vi "Particles_Setting_UI.vi"(4 "ForCalCalculaton In":T1, 6 "Analysis_Setting IN":T2={"PreProcess"=enum."*Algorithm*", "Parameter"=""}, 8 "error in (no error)":errorcluster, 9 "ProjectName":string, 10 "ROI List IN":refnum<vi>, 11 "Vision_Image":T1(plugin-control)) -> (0 "error out":errorcluster, 1 "Cancel?":bool, 2 "TempAnalysisResult":variant, 3 "Analysis_Setting":T2={"PreProcess"=enum."*Algorithm*", "Parameter"=""})   [LabVIEW 2019]
uses:
  Controls/_UI Command Cluster/Particle_UI Command Cluster.ctl
  Controls/Analysis_Type.ctl
  Controls/Analysis_Setting.ctl
  Controls/Particle/Analysis_Particle_Parameter.ctl
  <vilib>/vision/NI_Vision_Development_Module.lvlib
  Controls/V_Analysis_Type.ctl
  <vilib>/vision/Image Controls.llb/IMAQ Image.ctl
  Ctrl/VisionProcessName.ctl
panel:
  in  "Selected Particle":i32=2 min=-1 max=34
  in  "Simulation":bool
  out "Numeric":i32
  in  "Done":bool caption="完成"
  in  "Particle_UI Command":T4(ring)
  in  "Cancel":bool caption="取消"
  in  "ParticleTab":T5(tab)
  in  "MaxParticle":i32=1
  in  "Connectivity 4/8 (8)":bool=TRUE
  out "Selected Particle Report":T6(array[cluster]) {"Orientation" format="%.2f"; "Center of Mass"."Y" format="%.2f"; "Center of Mass"."X" format="%.2f"}
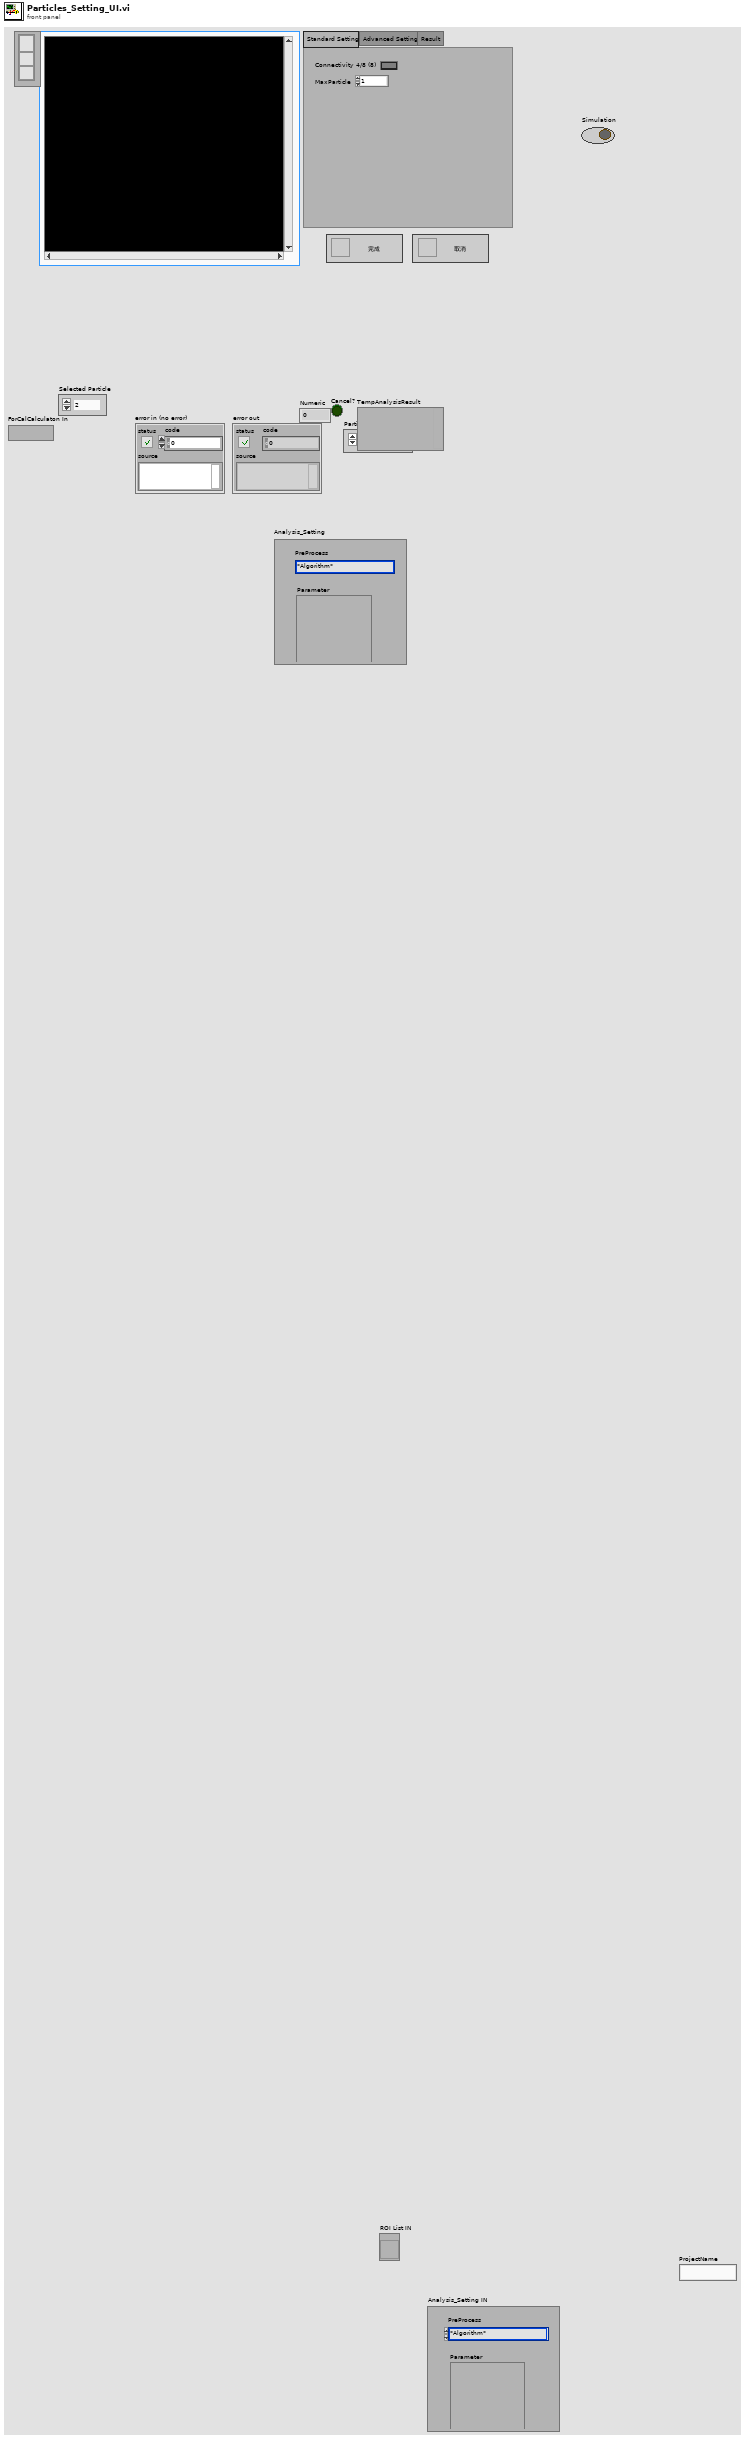
[diagram p1: front panel]
types:
  T1 = typedef "IMAQ Image.ctl" = refnum<image>
  T2 = typedef "Analysis_Setting.ctl" = cluster{"PreProcess":T3, "Parameter":string}
  T3 = typedef "VisionProcessName.ctl" = enum16{"*CamParameter*", "CamAttributes", "*Preprocess*", "CG_Brightness", "C_Plane Extraction", "C_Threshold", "G_Lookup Table", "G_Threshold", "B_Image Inversion", "*Algorithm*", "CG_Histogram", "C_Color Matching", "C_Color Pattern Matching", "G_PatternMatch", "CG_Find Straight Edge", "CG_Adv. Find Straight Edge", "CG_Find Circular Edge", "G_Max Clamp", "G_Clamp (Rake)", "G_Pattern Matching"}
  T4 = enum16{"Initialize", "Done", "Run Algorithm", "Cancel"}
  T5 = enum32{"Standard Setting", "Advanced Setting", "Result"}
  T6 = cluster{"Area":dbl, "Number of Holes":dbl, "Bounding Rect":cluster{"Left":dbl, "Top":dbl, "Right":dbl, "Bottom":dbl}, "Center of Mass":cluster{"X":dbl, "Y":dbl}, "Orientation":dbl, "Dimensions":cluster{"Width":dbl, "Height":dbl}}[]
  T7 = typedef "Particle_UI Command Cluster.ctl" = cluster{"Particle_UI Command":enum16{"Initialize", "Done", "Run Algorithm", "Cancel"}, "Selected Particle":i32, "Snap Simulation Mouse Down":bool, "Connectivity 4/8 (8)":bool, "MaxParticle":i32}
  T8 = typedef "IMAQ Line" = cluster{"Start X":i32, "Start Y":i32, "End X":i32, "End Y":i32}
  T9 = cluster{"Contour Type":u32, "ROI Type":u32, "Points":i32[]}
  T10 = typedef "Image Type" = u32
  T11 = typedef "Analysis_Particle_Parameter.ctl" = cluster{"Selected Particle":i32, "Connectivity 4/8 (8)":bool, "MaxParticle":i32}
  T12 = typedef "Analysis_Type.ctl" = u16
  T13 = typedef "ROI Descriptor" = cluster{"Global Rectangle":i32[], "Contours":cluster{"ID":enum32{"External", "Internal"}, "Type":u32, "Coordinates":i32[]}[]}
  T14 = typedef "Analysis_Setting.ctl" = cluster{"PreProcess":T15, "Parameter":string}
  T15 = typedef "V_Analysis_Type.ctl" = enum16{"None", "C_Color Pattern Matching", "G_PatternMatching", "G_ShapeDectect", "G_GeometricMatch", "B_Area Check"}
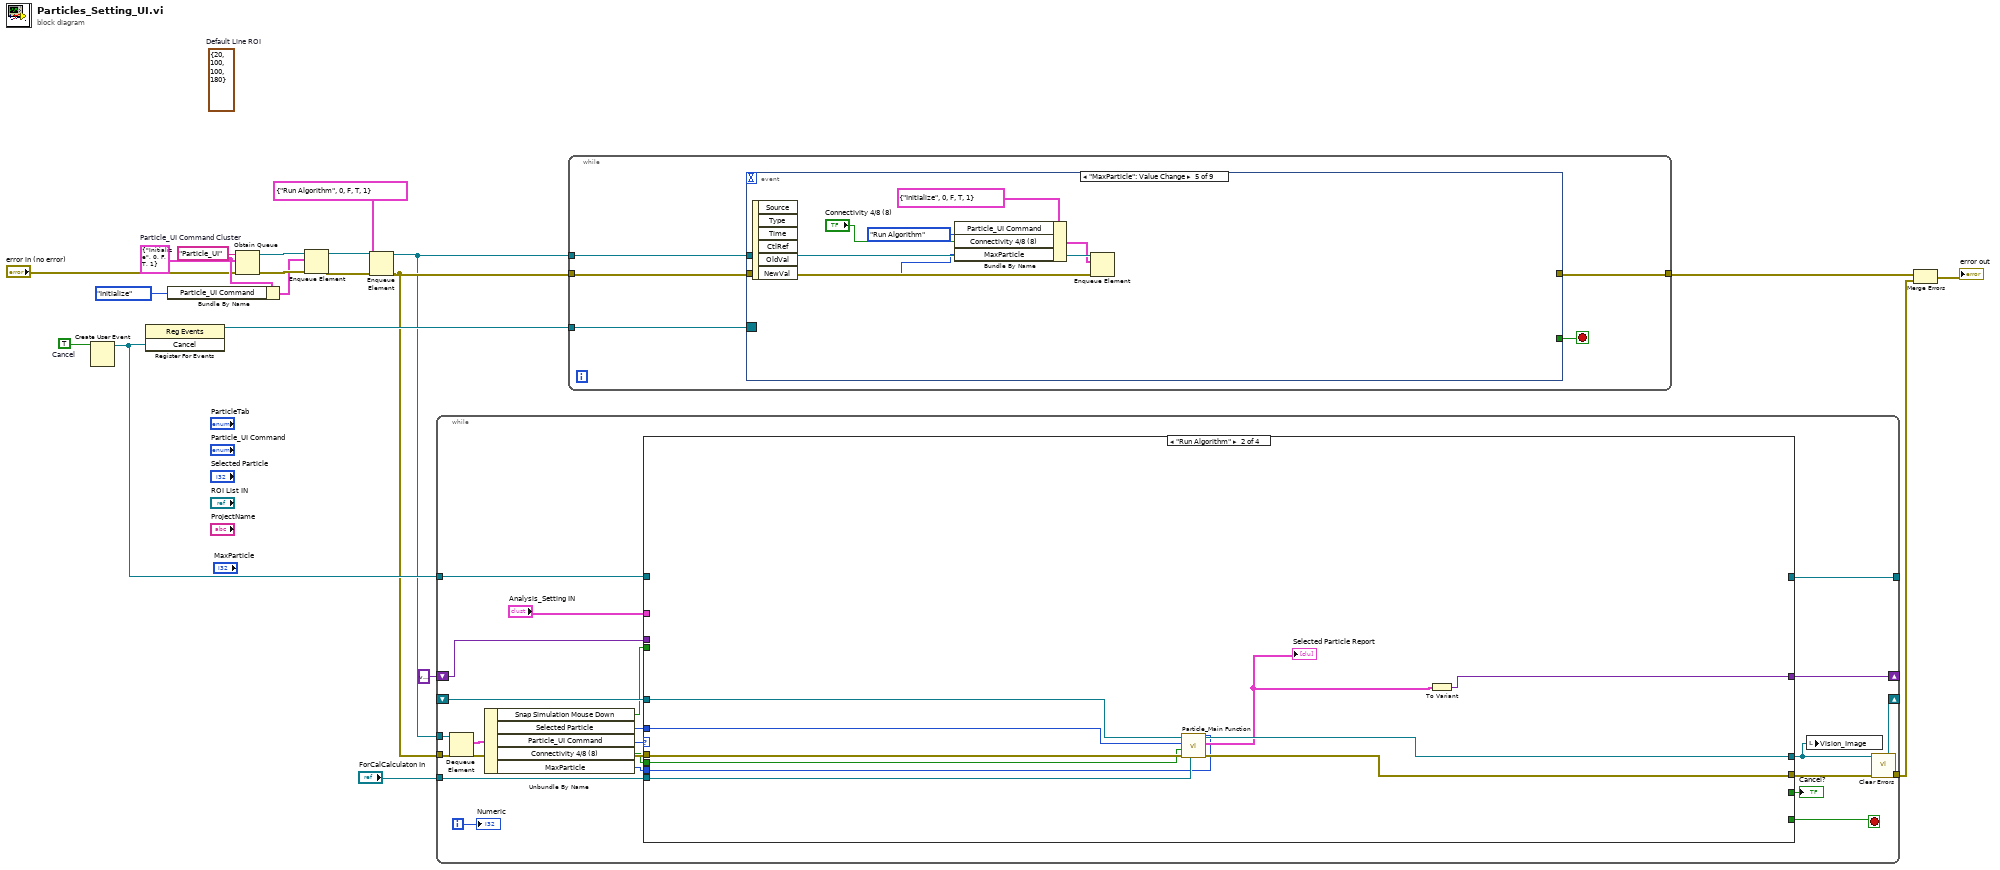
[diagram p0: block diagram]
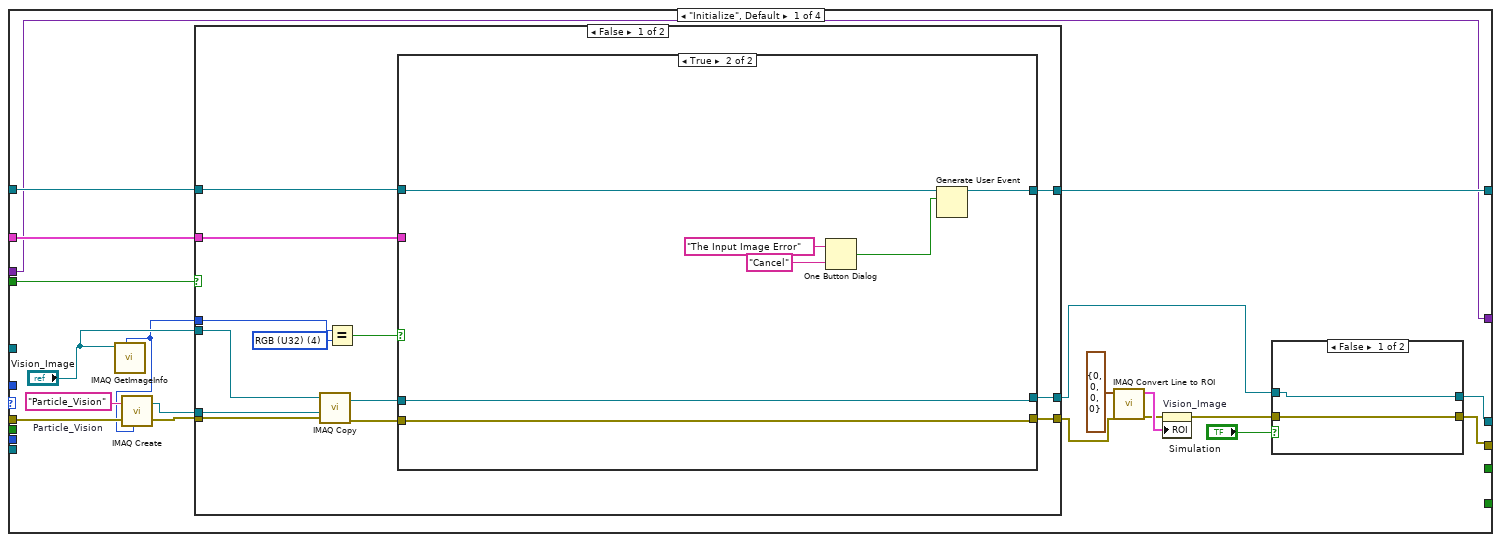
[diagram p2: hidden frame]
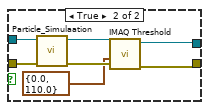
[diagram p3: hidden frame]
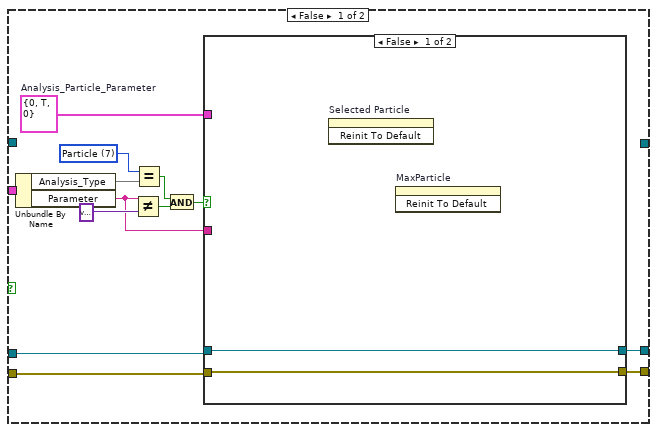
[diagram p4: hidden frame]
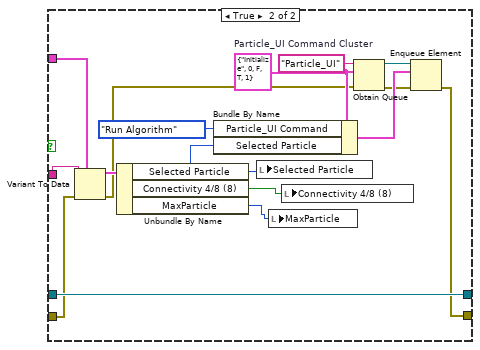
[diagram p5: hidden frame]
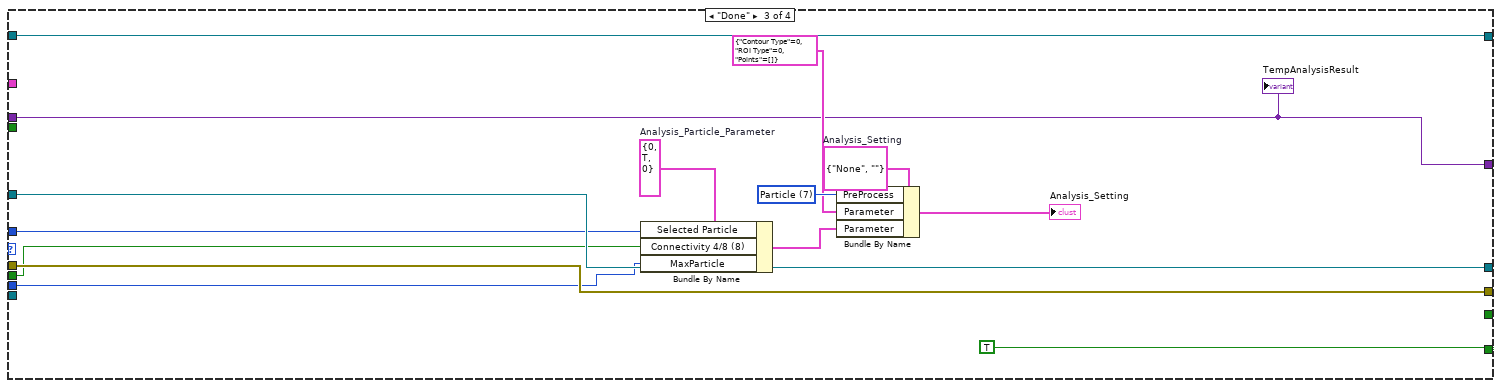
[diagram p7: hidden frame]
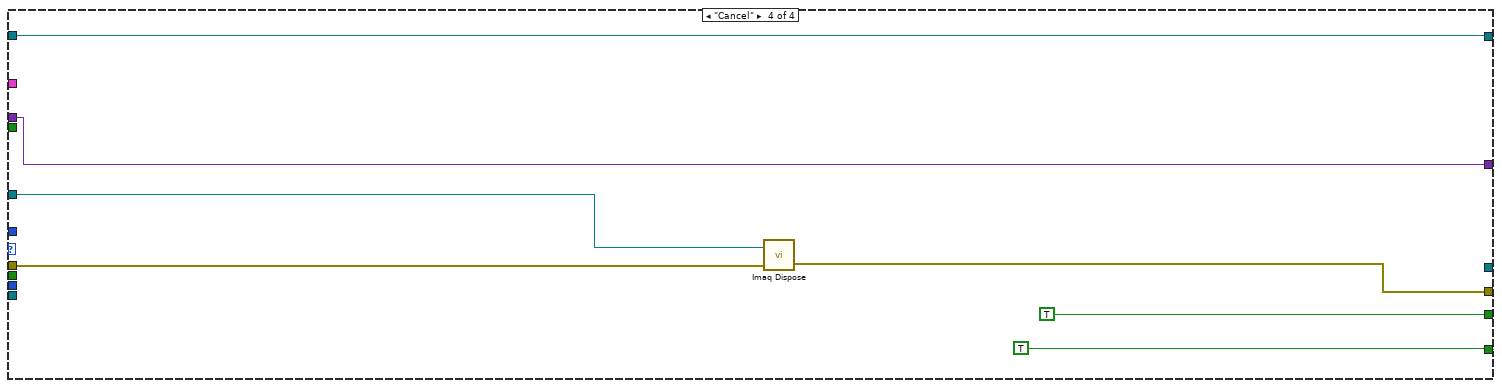
[diagram p8: hidden frame]
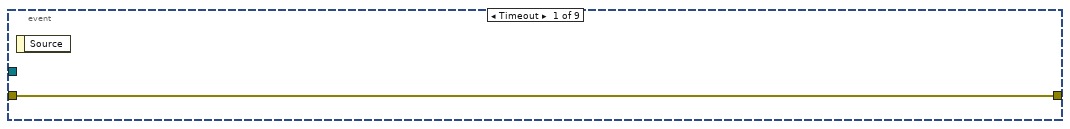
[diagram p9: hidden frame]
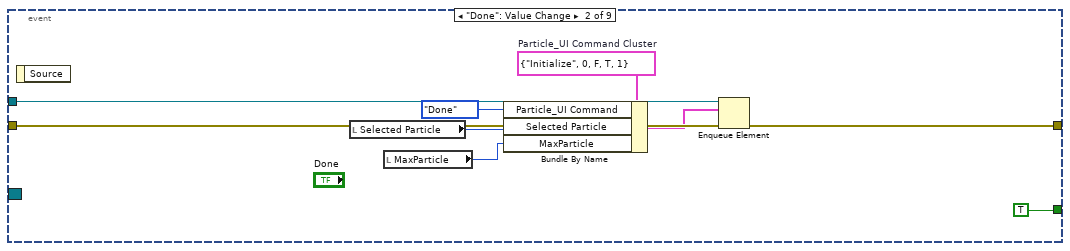
[diagram p10: hidden frame]
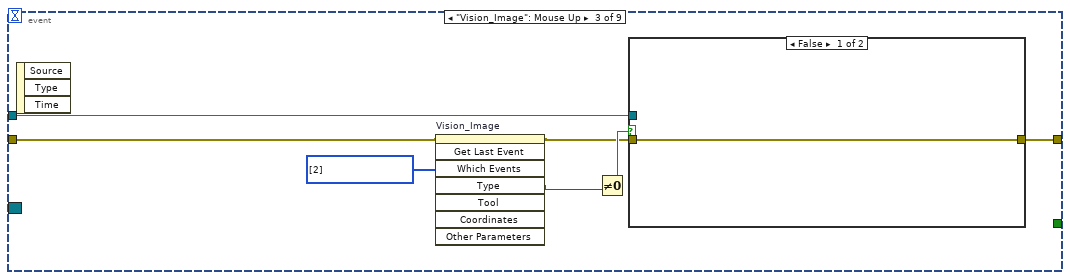
[diagram p11: hidden frame]
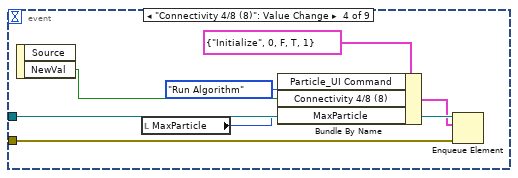
[diagram p13: hidden frame]
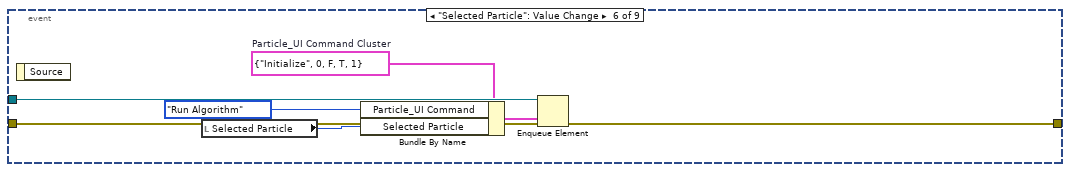
[diagram p14: hidden frame]
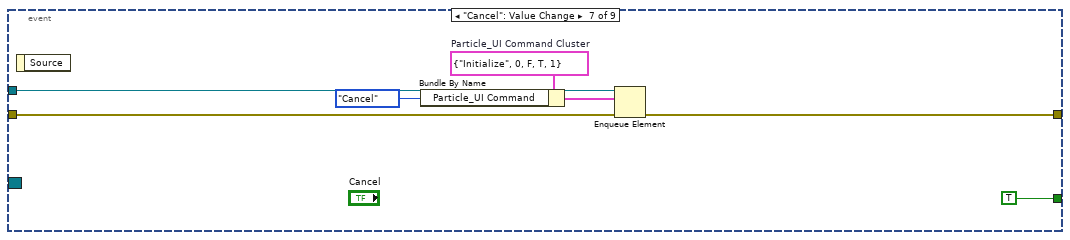
[diagram p15: hidden frame]
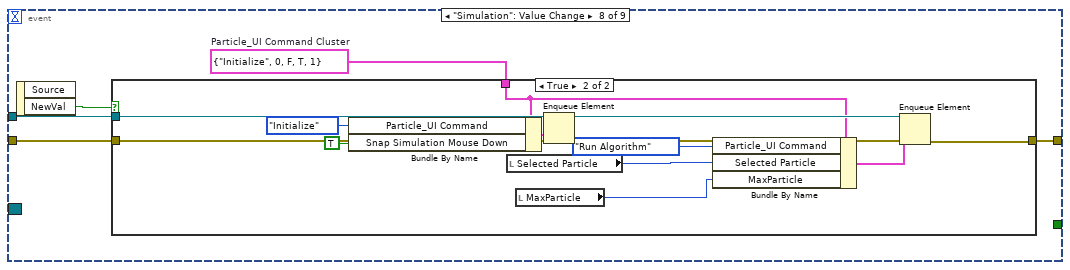
[diagram p16: hidden frame]
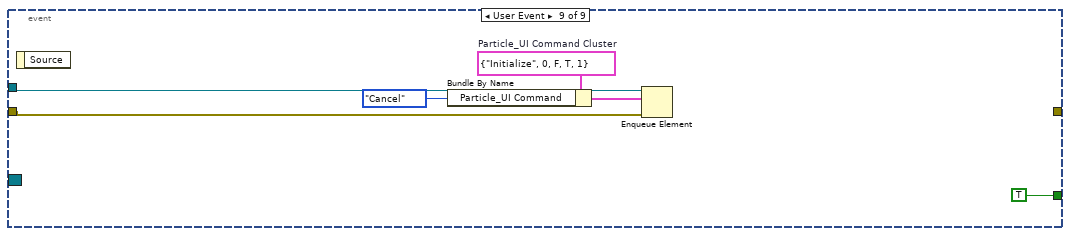
[diagram p18: hidden frame]
diagram:
  w10 = TRUE  # Cancel
  w13 = T7 {"Particle_UI Command"=enum."Initialize", "Selected Particle"=0, "Snap Simulation Mouse Down"=FALSE, "Connectivity 4/8 (8)"=TRUE, "MaxParticle"=1}  # Particle_UI Command Cluster
  (unwired) T8 {"Start X"=20, "Start Y"=100, "End X"=100, "End Y"=180}  # Default Line ROI
  n1 = Create User Event(user event datatype=w10) -> (user event=w8:refnum<user-event>)  [unwired: 1 in, 1 out]
  n2 = register-events(w8) -> (reference out=w9:refnum<event-registration>)  [unwired: 2 in, 1 out]
  n3 = Bundle By Name(cluster=w13, "Particle_UI Command"=T4."Initialize" ("Barcode 1D_UI Command")) -> (w14:T7)
  n4 = Obtain Queue(name (unnamed)="Particle_UI", element data type=w13, error in (no error)="error in (no error)") -> (queue out=w20:refnum<queue>, error out=w19:errorcluster)  [unwired: 2 in, 1 out]
  n5 = Enqueue Element(queue=w20, element=w14, error in (no error)=w19) -> (queue out=w5:refnum<queue>, error out=w7:errorcluster)  [unwired: 1 in, 1 out]
  n6 = Enqueue Element(queue=w5, element=T7 {"Particle_UI Command"=enum."Run Algorithm", "Selected Particle"=0, "Snap Simulation Mouse Down"=FALSE, "Connectivity 4/8 (8)"=TRUE, "MaxParticle"=1}, error in (no error)=w7) -> (queue out=w4:refnum<queue>, error out=w6:errorcluster)  [unwired: 1 in, 1 out]
  n7 = while {
    tunnel: w4 -> [w42]
    tunnel: w6 -> [w41]
    shift-right: [w34] -> _
    shift-left: _ -> [w36]
    tunnel: [w22] -> w16
    tunnel: w8 -> [w29]
    tunnel: [w28] -> _
    shift-right: [w27] -> _
    shift-left: variant ("Variant") -> [w26]
    tunnel: "ForCalCalculaton In" -> [w24]
    i -> [w35]
    stop <- w37 stop-if-true
    n8 = Dequeue Element(queue=w42, error in (no error)=w41) -> (element=w38:T7, error out=w39:errorcluster)  [unwired: 1 in, 2 out]
    n9 = Unbundle By Name(w38) -> ("Snap Simulation Mouse Down"=w30:bool, "Selected Particle"=w32:i32, "Particle_UI Command"=w40:T4, "Connectivity 4/8 (8)"=w25:bool, "MaxParticle"=w23:i32)
    n10 = case shown="\"Run Algorithm\"" w40 {
      tunnel: w39 -> [w61 w134 w146 w153]
      tunnel: [w48 w130 w146 w152] -> w21
      tunnel: [_ _ TRUE TRUE] -> w37
      tunnel: [w49 w131 w147 _] -> w34
      tunnel: w36 -> [_ w132 w147 w154]
      tunnel: [_ _ _ TRUE] -> w33
      tunnel: w32 -> [_ w133 w140 _]
      tunnel: "Analysis_Setting IN" -> [w60 _ _ _]
      tunnel: w30 -> [w52 _ _ _]
      tunnel: w29 -> [w47 _ w138 w150]
      tunnel: [w46 _ w138 w150] -> w28
      tunnel: [w43 w128 w137 w149] -> w27
      tunnel: w26 -> [w43 _ w137 w149]
      tunnel: w25 -> [_ w127 w136 _]
      tunnel: w24 -> [_ w126 _ _]
      tunnel: w23 -> [_ w125 w135 _]
      frame "Initialize", Default {
        w62 = "Particle_Vision"  # Particle_Vision
        n11 = call "IMAQ GetImageInfo"("Image"="Vision_Image") -> ("Image Type"=w44:T10)  [unwired: 3 in, 7 out]
        n12 = call "IMAQ Create"("Image Name"=w62, "Image Type"=w44, "error in (no error)"=w61) -> ("New Image"=w50:T1, "error out"=w51:errorcluster)  [unwired: 2 in]
        n13 = case shown="False" w52 {
          tunnel: w60 -> [w84 _]
          tunnel: [w83 w124] -> w53
          tunnel: [w82 w123] -> w54
          tunnel: w51 -> [w81 w123]
          tunnel: w50 -> [w80 w124]
          tunnel: w47 -> [w75 _]
          tunnel: [w74 _] -> w46
          tunnel: "Vision_Image" -> [w73 _]
          tunnel: w44 -> [w72 _]
          frame False {
            w77 = T10 4 items=["Grayscale (U8)", "Grayscale (I16)", "Grayscale (SGL)", "Complex (CSG)", "RGB (U32)", "HSL (U32)", "RGB (U64)", "Grayscale (U16)"] ("y")
            n14 = call "IMAQ Copy"("error in (no error)"=w81, "Image Dst"=w80, "Image Src"=w73) -> ("error out"=w79:errorcluster, "Image Dst Out"=w78:T1)  [unwired: 3 in]
            n15 = Equal?(x=w72, y=w77) -> (x = y?=w76:bool)
            n16 = case shown="True" w76 {
              tunnel: w84 -> [w90 _]
              tunnel: [w88 w116] -> w83
              tunnel: [w87 w117] -> w82
              tunnel: w79 -> [w86 w117]
              tunnel: w78 -> [w85 w116]
              tunnel: w75 -> [_ w119]
              tunnel: [_ w118] -> w74
              frame False {
                w89 = T11 {"Selected Particle"=0, "Connectivity 4/8 (8)"=TRUE, "MaxParticle"=0}  # Analysis_Particle_Parameter
                w95 = T12 7 items=["None", "PatternMatch", "Edge Detection", "Barcode 1D", "Barcode 2D", "Clamp", "Clamp MAX", "Particle", "Histogram", "Straight Edge", "Circle", "Shape Detect", "OCR", "Contour", "ColorMatch"] ("x")
                n17 = Unbundle By Name(w90) -> ("Analysis_Type"=w94, "Parameter"=w91:string)
                n18 = Not Equal?(x=w91, y=variant) -> (x != y?=w96:bool)
                n19 = Equal?(x=w95, y=w94) -> (x = y?=w97:bool)
                n20 = And(x=w97, y=w96) -> (x .and. y?=w92:bool)
                n21 = case shown="False" w92 {
                  tunnel: w86 -> [w98 w104]
                  tunnel: w85 -> [w99 w105]
                  tunnel: [w99 w105] -> w88
                  tunnel: [w98 w102] -> w87
                  tunnel: w91 -> [_ w115]
                  tunnel: w89 -> [_ w113]
                  frame False {
                    n22 = invoke on="Selected Particle" class="DigNum (strict)" method="Reinit To Default"() -> ()  [unwired: 3 in, 3 out]
                    n23 = invoke on="MaxParticle" class="DigNum (strict)" method="Reinit To Default"() -> ()  [unwired: 3 in, 3 out]
                  }
                  frame True {
                    w112 = T7 {"Particle_UI Command"=enum."Initialize", "Selected Particle"=0, "Snap Simulation Mouse Down"=FALSE, "Connectivity 4/8 (8)"=TRUE, "MaxParticle"=1}  # Particle_UI Command Cluster
                    n24 = Variant To Data(error in=w104, type=w113, Variant=w115) -> (data=w114:T11, error out=w103:errorcluster)
                    n25 = Unbundle By Name(w114) -> ("Selected Particle"=w106:i32, "Connectivity 4/8 (8)"=w101:bool, "MaxParticle"=w100:i32)
                    n26 = Bundle By Name(cluster=w112, "Particle_UI Command"=T4."Run Algorithm" ("Barcode 1D_UI Command"), "Selected Particle"=w106) -> (w111:T7)
                    n27 = local write "Selected Particle"(w106) -> ()
                    n28 = local write "MaxParticle"(w100) -> ()
                    n29 = local write "Connectivity 4/8 (8)"(w101) -> ()
                    n30 = Obtain Queue(name (unnamed)="Particle_UI", element data type=w112, error in (no error)=w103) -> (queue out=w107:refnum<queue>, error out=w108:errorcluster)  [unwired: 2 in, 1 out]
                    n31 = Enqueue Element(queue=w107, element=w111, error in (no error)=w108) -> (error out=w102:errorcluster)  [unwired: 1 in, 2 out]
                  }
                }
              }
              frame True {
                n32 = One Button Dialog(message="The Input Image Error", button name ("OK")="Cancel") -> (true=w120:bool)
                n33 = Generate User Event(user event=w119, event data cluster=w120) -> (user event out=w118:refnum<user-event>)  [unwired: 2 in, 1 out]
              }
            }
          }
          frame True {
          }
        }
        n34 = call "IMAQ Convert Line to ROI"("error in (no error)"=w54, "Line"=T8 {"Start X"=0, "Start Y"=0, "End X"=0, "End Y"=0}) -> ("error out"=w55:errorcluster, "ROI Descriptor"=w56:T13)  [unwired: 7 in]
        n35 = property on="Vision_Image" class="ImageControl"(error in=w55, "ROI"=w56) -> (error out=w58:errorcluster)  [unwired: 1 in, 1 out]
        n36 = case shown="False" "Simulation" {
          tunnel: [w64 w66] -> w48
          tunnel: [w63 w67] -> w49
          tunnel: w58 -> [w64 w71]
          tunnel: w53 -> [w63 w70]
          frame False {
          }
          frame True {
            n37 = call "Particle_Simulaation.vi"("error in (no error)"=w71, "Refnum in"=w70) -> ("error out"=w68:errorcluster, "Refnum out"=w69:T1)  [unwired: 8 in]
            n38 = call "IMAQ Threshold"("error in (no error)"=w68, "Range"=cluster{"Lower value":sgl, "Upper value":sgl} {"Lower value"=0.0, "Upper value"=110.0}, "Image Src"=w69) -> ("error out"=w66:errorcluster, "Image Dst Out"=w67:T1)  [unwired: 7 in]
          }
        }
      }
      frame "Run Algorithm" {
        n39 = call "Particle_Main Function.vi"("ForCalCalculaton In"=w126, "MAXParticle"=w125, "error in (no error)"=w134, "Connectivity 4/8 (8)"=w127, "Selected Particle"=w133, "Refnum in"=w132) -> ("error out"=w130:errorcluster, "Particle Report"=w129:T6, "Refnum out"=w131:T1)  [unwired: 1 in, 2 out]
        "Selected Particle Report" <- w129
        n40 = To Variant(anything=w129) -> (Variant=w128:variant)
      }
      frame "Done" {
        w142 = T11 {"Selected Particle"=0, "Connectivity 4/8 (8)"=TRUE, "MaxParticle"=0}  # Analysis_Particle_Parameter
        w144 = T12 7 items=["None", "PatternMatch", "Edge Detection", "Barcode 1D", "Barcode 2D", "Clamp", "Clamp MAX", "Particle", "Histogram", "Straight Edge", "Circle", "Shape Detect", "OCR", "Contour", "ColorMatch"] ("Analysis_Type")
        w145 = T14 {"PreProcess"=enum."None", "Parameter"=""}  # Analysis_Setting
        n41 = Bundle By Name(cluster=w142, "Selected Particle"=w140, "Connectivity 4/8 (8)"=w136, "MaxParticle"=w135) -> (w141:T11)
        n42 = Bundle By Name(cluster=w145, "PreProcess"=w144, "Parameter"=T9 {"Contour Type"=0, "ROI Type"=0, "Points"=[]} ("RegionContour"), "Parameter"=w141) -> (→"Analysis_Setting":T14)
        "TempAnalysisResult" <- w137
      }
      frame "Cancel" {
        n43 = call "Imaq Dispose"("Image"=w154, "error in (no error)"=w153) -> ("error out"=w152:errorcluster)  [unwired: 4 in]
      }
    }
    "Cancel?" <- w33
    n44 = local write "Vision_Image"(w34) -> ()
    n45 = call <vilib>:"Clear Errors.vi"("error in (no error)"=w21) -> ("error out"=w22:errorcluster)  [unwired: 5 in, 1 out]
    "Numeric" <- w35
  }
  n46 = while {
    tunnel: w4 -> [w160]
    tunnel: w6 -> [w159]
    tunnel: [w157] -> w17
    tunnel: w9 -> [w156]
    stop <- w158 stop-if-true
    n47 = event shown="[4] \"MaxParticle\": Value Change" {
      selector: w156 -> [_ _ _ _ _ _ _ _ _]
      dyn-events: _ -> [_ _ _ _ _ _ _ _ _]
      timeout: _ -> [_ _ _ _ _ _ _ _ _]
      tunnel: w160 -> [_ w170 w177 w186 w193 w200 w207 w212 w228]
      tunnel: w159 -> [w161 w169 w174 w185 w192 w199 w206 w211 w227]
      tunnel: [_ TRUE _ _ _ _ TRUE _ TRUE] -> w158
      tunnel: [w161 w168 w171 _ _ w198 w204 w209 _] -> w157
      event Timeout {
        n48 = event-data() -> ()  [unwired: 1 in, 1 out]
      }
      event "Done": Value Change {
        w167 = T7 {"Particle_UI Command"=enum."Initialize", "Selected Particle"=0, "Snap Simulation Mouse Down"=FALSE, "Connectivity 4/8 (8)"=TRUE, "MaxParticle"=1}  # Particle_UI Command Cluster
        n49 = event-data() -> ()  [unwired: 1 in, 1 out]
        n50 = local read "Selected Particle"() -> (w163:i32)
        n51 = local read "MaxParticle"() -> (w162:i32)
        n52 = Bundle By Name(cluster=w167, "Particle_UI Command"=T4."Done" ("Edge Detection_UI Command"), "Selected Particle"=w163, "MaxParticle"=w162) -> (w165:T7)
        n53 = Enqueue Element(queue=w170, element=w165, error in (no error)=w169) -> (error out=w168:errorcluster)  [unwired: 1 in, 2 out]
      }
      event "Vision_Image": Mouse Up {
        w175 = i32[] [2] items=["No Event"=0, "Click Event"=1, "Draw Event"=2, "Size Event"=4, "Scroll Event"=5, "Double Click Event"=8] ("Which Events")
        n54 = event-data() -> ()  [unwired: 1 in, 3 out]
        n55 = invoke on="Vision_Image" class="ImageControl" method="Get Last Event"(error in=w174, "Which Events"=w175) -> (error out=w173:errorcluster, "Type"=w172:i32)  [unwired: 6 in, 6 out]
        n56 = Not Equal To 0?(x=w172) -> (x != 0?=w176:bool)
        n57 = case shown="False" w176 {
          tunnel: w177 -> [_ _]
          tunnel: w173 -> [w178 w179]
          tunnel: [w178 w179] -> w171
          frame False {
          }
          frame True {
          }
        }
      }
      event "Connectivity 4/8 (8)": Value Change {
        n58 = event-data() -> ("NewVal"=w181:bool)  [unwired: 1 in, 1 out]
        n59 = local read "MaxParticle"() -> (w180:i32)
        n60 = Bundle By Name(cluster=T7 {"Particle_UI Command"=enum."Initialize", "Selected Particle"=0, "Snap Simulation Mouse Down"=FALSE, "Connectivity 4/8 (8)"=TRUE, "MaxParticle"=1} ("element"), "Particle_UI Command"=T4."Run Algorithm", "Connectivity 4/8 (8)"=w181, "MaxParticle"=w180) -> (w183:T7)
        n61 = Enqueue Element(queue=w186, element=w183, error in (no error)=w185) -> ()  [unwired: 1 in, 3 out]
      }
      event "MaxParticle": Value Change {
        n62 = event-data() -> ("NewVal"=w188:i32)  [unwired: 1 in, 5 out]
        n63 = Bundle By Name(cluster=T7 {"Particle_UI Command"=enum."Initialize", "Selected Particle"=0, "Snap Simulation Mouse Down"=FALSE, "Connectivity 4/8 (8)"=TRUE, "MaxParticle"=1} ("element"), "Particle_UI Command"=T4."Run Algorithm", "Connectivity 4/8 (8)"="Connectivity 4/8 (8)", "MaxParticle"=w188) -> (w190:T7)
        n64 = Enqueue Element(queue=w193, element=w190, error in (no error)=w192) -> ()  [unwired: 1 in, 3 out]
      }
      event "Selected Particle": Value Change {
        w197 = T7 {"Particle_UI Command"=enum."Initialize", "Selected Particle"=0, "Snap Simulation Mouse Down"=FALSE, "Connectivity 4/8 (8)"=TRUE, "MaxParticle"=1}  # Particle_UI Command Cluster
        n65 = event-data() -> ()  [unwired: 1 in, 1 out]
        n66 = local read "Selected Particle"() -> (w194:i32)
        n67 = Bundle By Name(cluster=w197, "Particle_UI Command"=T4."Run Algorithm" ("Barcode 1D_UI Command"), "Selected Particle"=w194) -> (w195:T7)
        n68 = Enqueue Element(queue=w200, element=w195, error in (no error)=w199) -> (error out=w198:errorcluster)  [unwired: 1 in, 2 out]
      }
      event "Cancel": Value Change {
        w202 = T7 {"Particle_UI Command"=enum."Initialize", "Selected Particle"=0, "Snap Simulation Mouse Down"=FALSE, "Connectivity 4/8 (8)"=TRUE, "MaxParticle"=1}  # Particle_UI Command Cluster
        n69 = event-data() -> ()  [unwired: 1 in, 1 out]
        n70 = Bundle By Name(cluster=w202, "Particle_UI Command"=T4."Cancel" ("Barcode 1D_UI Command")) -> (w201:T7)
        n71 = Enqueue Element(queue=w207, element=w201, error in (no error)=w206) -> (error out=w204:errorcluster)  [unwired: 1 in, 2 out]
      }
      event "Simulation": Value Change {
        w208 = T7 {"Particle_UI Command"=enum."Initialize", "Selected Particle"=0, "Snap Simulation Mouse Down"=FALSE, "Connectivity 4/8 (8)"=TRUE, "MaxParticle"=1}  # Particle_UI Command Cluster
        n72 = event-data() -> ("NewVal"=w210:bool)  [unwired: 1 in, 1 out]
        n73 = case shown="True" w210 {
          tunnel: w212 -> [_ w226]
          tunnel: w211 -> [w213 w225]
          tunnel: w208 -> [_ w219]
          tunnel: [w213 w220] -> w209
          frame False {
          }
          frame True {
            n74 = Bundle By Name(cluster=w219, "Particle_UI Command"=T4."Initialize" ("Barcode 1D_UI Command"), "Snap Simulation Mouse Down"=TRUE) -> (w223:T7)
            n75 = local read "Selected Particle"() -> (w216:i32)
            n76 = local read "MaxParticle"() -> (w214:i32)
            n77 = Enqueue Element(queue=w226, element=w223, error in (no error)=w225) -> (queue out=w222:refnum<queue>, error out=w221:errorcluster)  [unwired: 1 in, 1 out]
            n78 = Bundle By Name(cluster=w219, "Particle_UI Command"=T4."Run Algorithm", "Selected Particle"=w216, "MaxParticle"=w214) -> (w218:T7)
            n79 = Enqueue Element(queue=w222, element=w218, error in (no error)=w221) -> (error out=w220:errorcluster)  [unwired: 1 in, 2 out]
          }
        }
      }
      event User Event {
        w230 = T7 {"Particle_UI Command"=enum."Initialize", "Selected Particle"=0, "Snap Simulation Mouse Down"=FALSE, "Connectivity 4/8 (8)"=TRUE, "MaxParticle"=1}  # Particle_UI Command Cluster
        n80 = event-data() -> ()  [unwired: 1 in, 1 out]
        n81 = Bundle By Name(cluster=w230, "Particle_UI Command"=T4."Cancel" ("Barcode 1D_UI Command")) -> (w229:T7)
        n82 = Enqueue Element(queue=w228, element=w229, error in (no error)=w227) -> ()  [unwired: 1 in, 3 out]
      }
    }
  }
  n83 = Merge Errors(w17, w16) -> (→"error out":errorcluster)
